vi "New JSON Boolean.vi"(8 "error in (no error)":errorcluster, 10 "value":bool) -> (0 "error out":errorcluster, 3 "JSON Value out":refnum<class "JSON Value.lvclass">)   [LabVIEW 2016, in "JSON Value.lvclass"]
doc: "Creates a new JSON Boolean initialized with the given value"
uses:
  JSON Value.lvclass
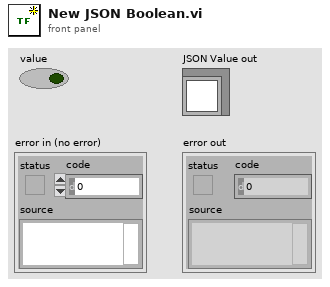
[diagram p1: front panel]
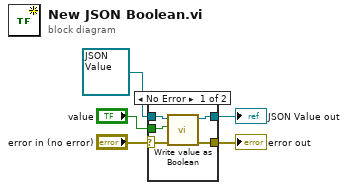
[diagram p0: block diagram]
diagram:
  n1 = case shown="No Error" "error in (no error)" {
    selector: "error in (no error)" -> [w7 w12]
    tunnel: [w9 w12] -> w4
    tunnel: [w10 w11] -> w3
    tunnel: refnum<class "JSON Value.lvclass"> refnum ("JSON out") -> [w8 w11]
    tunnel: "value" -> [w6 _]
    frame No Error {
      n2 = call "Write value as Boolean.vi"("error in (no error)"=w7, "value"=w6, "JSON Value in"=w8) -> ("error out"=w9:errorcluster, "JSON Value out"=w10:refnum<class "JSON Value.lvclass">)  [unwired: 7 in]
    }
    frame Error {
    }
  }
  "error out" <- w4
  "JSON Value out" <- w3
